vi "fita2_D.vi"() -> ()   [LabVIEW 2014]
uses:
  <vilib>/Analysis/5stat.llb/RMS (DBL).vi
  <vilib>/DAQmx/create/channels.llb/DAQmx Create Channel (AI-Voltage-Basic).vi
  <vilib>/DAQmx/configure/timing.llb/DAQmx Timing (Sample Clock).vi
  <vilib>/DAQmx/read.llb/DAQmx Read (Analog 1D Wfm NChan NSamp).vi
  <vilib>/Waveform/WDTOps.llb/WDT Index Channel DBL.vi
  <vilib>/Utility/file.llb/Write To Spreadsheet File (string).vi
  <vilib>/Analysis/NI_AALPro.lvlib
panel:
  out "CH4":dbl
  out "CH3":dbl
  out "CH2":dbl
  out "CH1":dbl
  out "MIN CH4":bool
  out "MIN CH2":bool
  out "MIN CH1":bool
  out "MIN CH3":bool
  out "MAX CH4":bool
  out "MAX CH3":bool
  out "MAX CH2":bool
  out "MAX CH1":bool
  in  "Temp Max CH2":dbl
  in  "Temp Min CH1":dbl
  in  "Temp Min CH2":dbl
  in  "Temp Max CH3":dbl
  in  "Temp Min CH3":dbl
  in  "Temp Max CH4":dbl
  in  "Temp Min CH4":dbl
  in  "Temp Max CH1":dbl
  in  "Start":bool
  in  "stop":bool
  out "Waveform Chart":T1(graph)
  out "Canals seleccionats":dbl
  in  "Durada adquisicio":dbl
  in  "Temps entre adquisicio":dbl
  in  "Numero de mostres per fer mitja":u32
  in  "Nombre de Canals":string(combo)
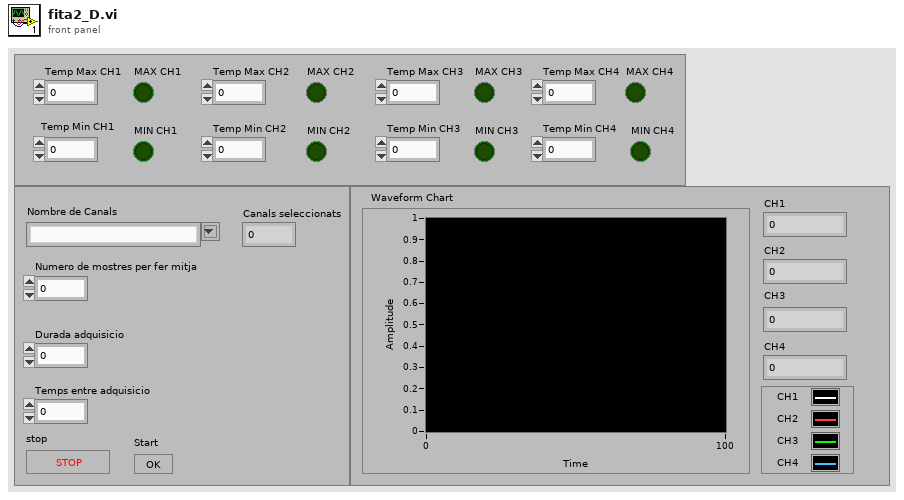
[diagram p1: front panel]
types:
  T1 = cluster{"rms value":dbl, "rms value":dbl, "rms value":dbl, "rms value":dbl}
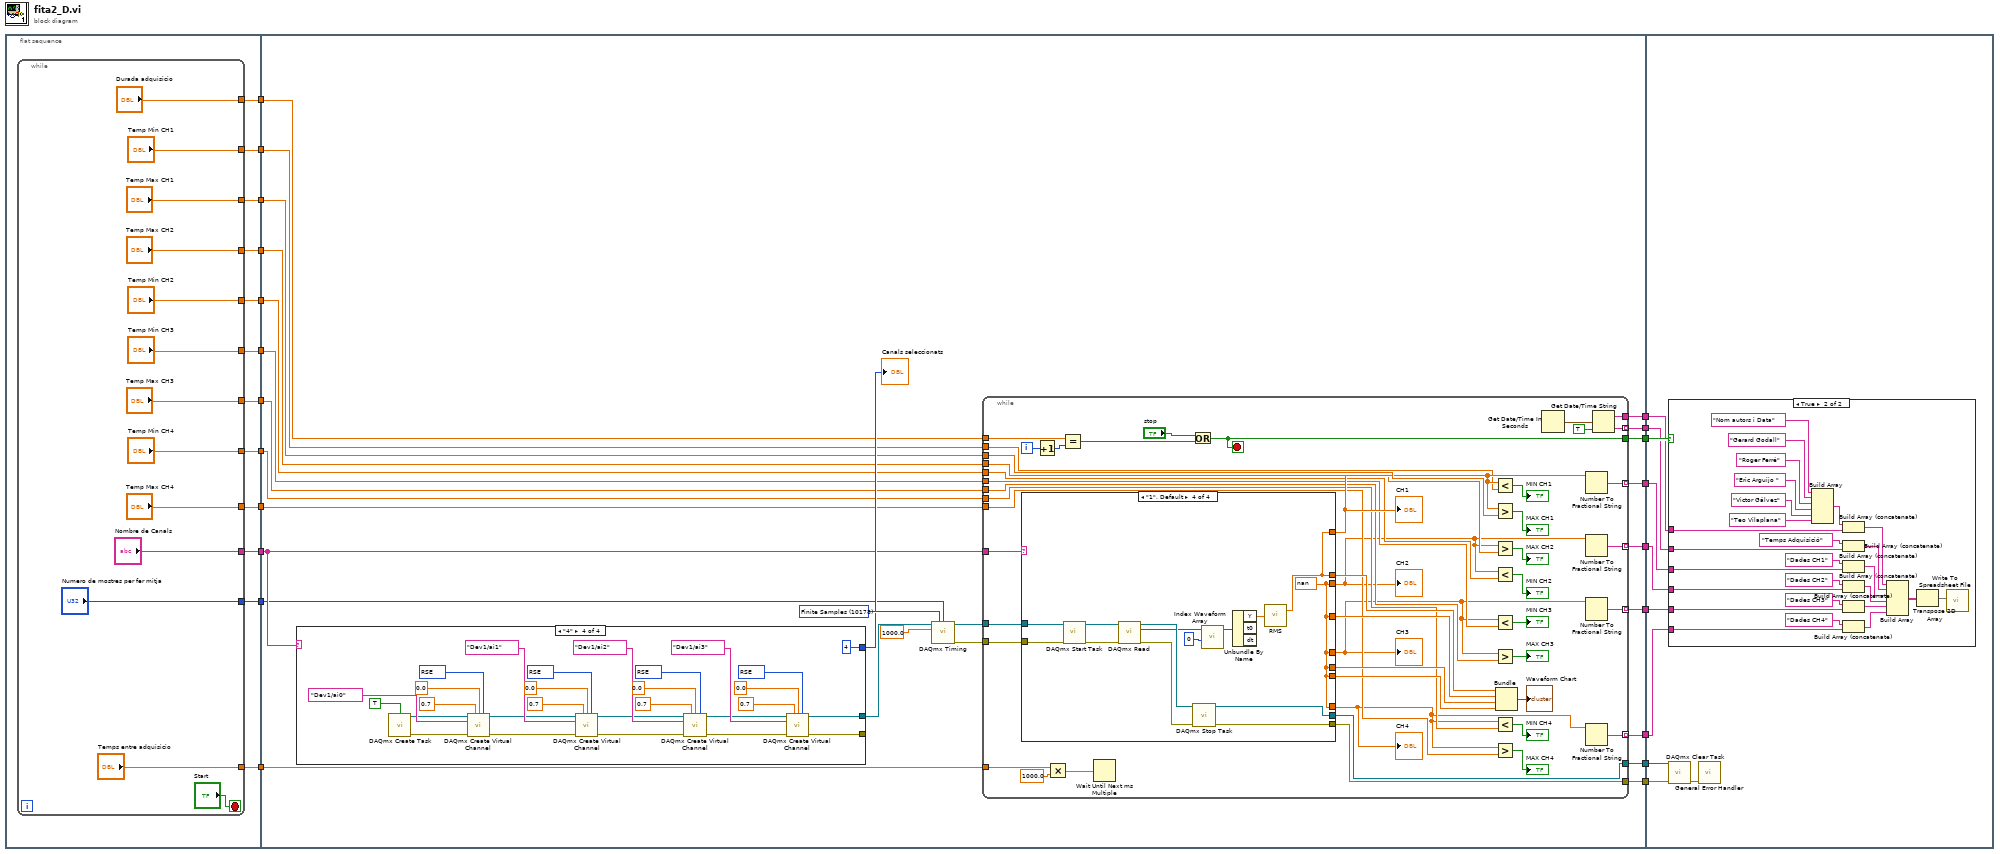
[diagram p0: block diagram]
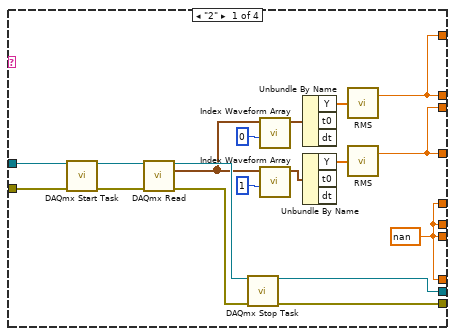
[diagram p2: hidden frame]
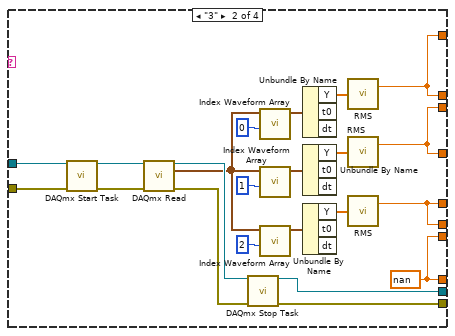
[diagram p3: hidden frame]
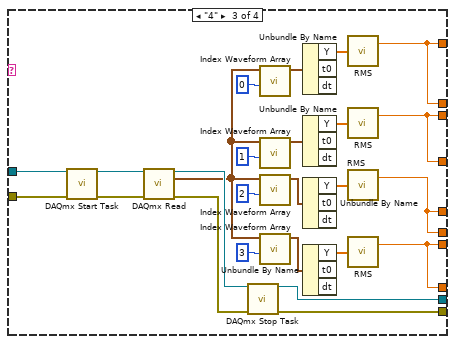
[diagram p4: hidden frame]
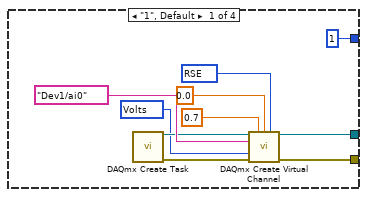
[diagram p5: hidden frame]
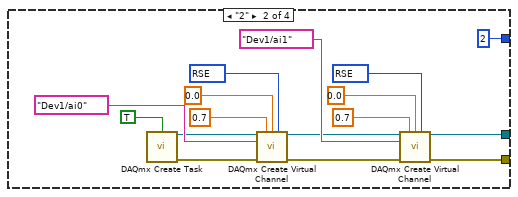
[diagram p6: hidden frame]
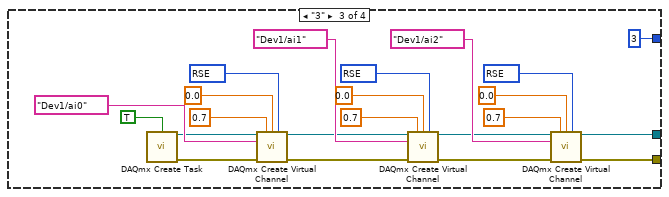
[diagram p7: hidden frame]
diagram:
  n1 = flat-sequence {
    tunnel: [w33] -> w21
    tunnel: [w32] -> w20
    tunnel: [w31] -> w19
    tunnel: [w30] -> w18
    tunnel: [w29] -> w13
    tunnel: [w28] -> w12
    tunnel: [w27] -> w11
    tunnel: [w26] -> w10
    tunnel: [w25] -> w9
    tunnel: [w24] -> w8
    tunnel: [w23] -> w7
    tunnel: [w22] -> w6
    tunnel: w21 -> [w67]
    tunnel: w20 -> [w66]
    tunnel: w19 -> [w65]
    tunnel: w18 -> [w64]
    tunnel: [w63] -> w17
    tunnel: [w62] -> w16
    tunnel: [w61] -> w15
    tunnel: [w60] -> w14
    tunnel: w13 -> [w59]
    tunnel: w12 -> [w58]
    tunnel: w11 -> [w57]
    tunnel: w10 -> [w56]
    tunnel: w9 -> [w55]
    tunnel: w8 -> [w54]
    tunnel: w7 -> [w53]
    tunnel: w6 -> [w52]
    tunnel: [w51] -> w5
    tunnel: [w50] -> w4
    tunnel: [w49] -> w3
    tunnel: [w48] -> w2
    tunnel: [w47] -> w1
    tunnel: w17 -> [w284]
    tunnel: w16 -> [w283]
    tunnel: w15 -> [w282]
    tunnel: w14 -> [w281]
    tunnel: w5 -> [w280]
    tunnel: w4 -> [w279]
    tunnel: w3 -> [w278]
    tunnel: w2 -> [w277]
    tunnel: w1 -> [w276]
    frame #0 {
      n2 = while {
        tunnel: ["Nombre de Canals"] -> w33
        tunnel: ["Durada adquisicio"] -> w32
        tunnel: ["Temps entre adquisicio"] -> w31
        tunnel: ["Numero de mostres per fer mitja"] -> w30
        tunnel: ["Temp Max CH1"] -> w29
        tunnel: ["Temp Min CH1"] -> w28
        tunnel: ["Temp Max CH3"] -> w27
        tunnel: ["Temp Max CH2"] -> w26
        tunnel: ["Temp Max CH4"] -> w25
        tunnel: ["Temp Min CH3"] -> w24
        tunnel: ["Temp Min CH2"] -> w23
        tunnel: ["Temp Min CH4"] -> w22
        stop <- "Start" stop-if-true
      }
    }
    frame #1 {
      w72 = 10178 items=["Finite Samples"=10178, "Continuous Samples"=10123, "Hardware Timed Single Point"=12522] ("sample mode")
      n3 = case shown="\"4\"" w67 {
        tunnel: [w203 w212 w228 w250] -> w73
        tunnel: [w202 w211 w227 w249] -> _
        tunnel: [1 2 3 4] -> w71
        frame "1", Default {
          w200 = 10348 items=["Volts"=10348, "From Custom Scale"=10065] ("units")
          w206 = 10083 items=["default"=-1, "RSE"=10083, "NRSE"=10078, "Differential"=10106, "Pseudodifferential"=12529] ("input terminal configuration")
          n4 = call <vilib>:"DAQmx Create Task.vi"() -> ("task out"=w204:refnum<k21>, "error out"=w205:errorcluster)  [unwired: 14 in]
          n5 = call-poly <vilib>:"DAQmx Create Virtual Channel.vi"("task in"=w204, "maximum value"=0.7, "minimum value"=0.0, "input terminal configuration"=w206, "physical channels"=tag "Dev1/ai0", "units"=w200, "error in"=w205) -> ("task out"=w203:refnum<k21>, "error out"=w202:errorcluster)  [unwired: 7 in]
        }
        frame "2" {
          w215 = 10083 items=["default"=-1, "RSE"=10083, "NRSE"=10078, "Differential"=10106, "Pseudodifferential"=12529] ("input terminal configuration")
          w222 = 10083 items=["default"=-1, "RSE"=10083, "NRSE"=10078, "Differential"=10106, "Pseudodifferential"=12529] ("input terminal configuration")
          n6 = call <vilib>:"DAQmx Create Task.vi"("auto cleanup"=TRUE) -> ("task out"=w220:refnum<k21>, "error out"=w221:errorcluster)  [unwired: 13 in]
          n7 = call-poly <vilib>:"DAQmx Create Virtual Channel.vi"("task in"=w220, "maximum value"=0.7, "minimum value"=0.0, "input terminal configuration"=w222, "physical channels"=tag "Dev1/ai0", "error in"=w221) -> ("task out"=w214:refnum<k21>, "error out"=w213:errorcluster)  [unwired: 8 in]
          n8 = call-poly <vilib>:"DAQmx Create Virtual Channel.vi"("task in"=w214, "maximum value"=0.7, "minimum value"=0.0, "input terminal configuration"=w215, "physical channels"=tag "Dev1/ai1", "error in"=w213) -> ("task out"=w212:refnum<k21>, "error out"=w211:errorcluster)  [unwired: 8 in]
        }
        frame "3" {
          w231 = 10083 items=["default"=-1, "RSE"=10083, "NRSE"=10078, "Differential"=10106, "Pseudodifferential"=12529] ("input terminal configuration")
          w237 = 10083 items=["default"=-1, "RSE"=10083, "NRSE"=10078, "Differential"=10106, "Pseudodifferential"=12529] ("input terminal configuration")
          w244 = 10083 items=["default"=-1, "RSE"=10083, "NRSE"=10078, "Differential"=10106, "Pseudodifferential"=12529] ("input terminal configuration")
          n9 = call <vilib>:"DAQmx Create Task.vi"("auto cleanup"=TRUE) -> ("task out"=w242:refnum<k21>, "error out"=w243:errorcluster)  [unwired: 13 in]
          n10 = call-poly <vilib>:"DAQmx Create Virtual Channel.vi"("task in"=w242, "maximum value"=0.7, "minimum value"=0.0, "input terminal configuration"=w244, "physical channels"=tag "Dev1/ai0", "error in"=w243) -> ("task out"=w236:refnum<k21>, "error out"=w235:errorcluster)  [unwired: 8 in]
          n11 = call-poly <vilib>:"DAQmx Create Virtual Channel.vi"("task in"=w236, "maximum value"=0.7, "minimum value"=0.0, "input terminal configuration"=w237, "physical channels"=tag "Dev1/ai1", "error in"=w235) -> ("task out"=w230:refnum<k21>, "error out"=w229:errorcluster)  [unwired: 8 in]
          n12 = call-poly <vilib>:"DAQmx Create Virtual Channel.vi"("task in"=w230, "maximum value"=0.7, "minimum value"=0.0, "input terminal configuration"=w231, "physical channels"=tag "Dev1/ai2", "error in"=w229) -> ("task out"=w228:refnum<k21>, "error out"=w227:errorcluster)  [unwired: 8 in]
        }
        frame "4" {
          w253 = 10083 items=["default"=-1, "RSE"=10083, "NRSE"=10078, "Differential"=10106, "Pseudodifferential"=12529] ("input terminal configuration")
          w259 = 10083 items=["default"=-1, "RSE"=10083, "NRSE"=10078, "Differential"=10106, "Pseudodifferential"=12529] ("input terminal configuration")
          w265 = 10083 items=["default"=-1, "RSE"=10083, "NRSE"=10078, "Differential"=10106, "Pseudodifferential"=12529] ("input terminal configuration")
          w272 = 10083 items=["default"=-1, "RSE"=10083, "NRSE"=10078, "Differential"=10106, "Pseudodifferential"=12529] ("input terminal configuration")
          n13 = call <vilib>:"DAQmx Create Task.vi"("auto cleanup"=TRUE) -> ("task out"=w270:refnum<k21>, "error out"=w271:errorcluster)  [unwired: 13 in]
          n14 = call-poly <vilib>:"DAQmx Create Virtual Channel.vi"("task in"=w270, "maximum value"=0.7, "minimum value"=0.0, "input terminal configuration"=w272, "physical channels"=tag "Dev1/ai0", "error in"=w271) -> ("task out"=w264:refnum<k21>, "error out"=w263:errorcluster)  [unwired: 8 in]
          n15 = call-poly <vilib>:"DAQmx Create Virtual Channel.vi"("task in"=w264, "maximum value"=0.7, "minimum value"=0.0, "input terminal configuration"=w265, "physical channels"=tag "Dev1/ai1", "error in"=w263) -> ("task out"=w258:refnum<k21>, "error out"=w257:errorcluster)  [unwired: 8 in]
          n16 = call-poly <vilib>:"DAQmx Create Virtual Channel.vi"("task in"=w258, "maximum value"=0.7, "minimum value"=0.0, "input terminal configuration"=w259, "physical channels"=tag "Dev1/ai2", "error in"=w257) -> ("task out"=w252:refnum<k21>, "error out"=w251:errorcluster)  [unwired: 8 in]
          n17 = call-poly <vilib>:"DAQmx Create Virtual Channel.vi"("task in"=w252, "maximum value"=0.7, "minimum value"=0.0, "input terminal configuration"=w253, "physical channels"=tag "Dev1/ai3", "error in"=w251) -> ("task out"=w250:refnum<k21>, "error out"=w249:errorcluster)  [unwired: 8 in]
        }
      }
      "Canals seleccionats" <- w71
      n18 = call-poly <vilib>:"DAQmx Timing.vi"("task/channels in"=w73, "sample mode"=w72, "samples per channel"=w64, "rate"=1000.0) -> ("task out"=w69:refnum<k21>, "error out"=w68:errorcluster)  [unwired: 10 in]
      n19 = while {
        tunnel: w65 -> [w118]
        tunnel: w67 -> [w117]
        tunnel: w69 -> [w116]
        tunnel: w68 -> [w115]
        tunnel: [w114] -> w63
        tunnel: [w113] -> w62
        tunnel: w66 -> [w104]
        tunnel: [w103] -> w61
        tunnel: [w101] -> w60 mode=indexing
        tunnel: w59 -> [w100]
        tunnel: w58 -> [w96]
        tunnel: w57 -> [w88]
        tunnel: w56 -> [w87]
        tunnel: w55 -> [w86]
        tunnel: w54 -> [w85]
        tunnel: w53 -> [w84]
        tunnel: w52 -> [w83]
        tunnel: [w81] -> w51 mode=indexing
        tunnel: [w79] -> w50 mode=indexing
        tunnel: [w77] -> w49 mode=indexing
        tunnel: [w76] -> w48
        tunnel: [w75] -> w47 mode=indexing
        i -> [w110]
        stop <- w103 stop-if-true
        n20 = case shown="\"1\", Default" w117 {
          tunnel: w116 -> [w127 w146 w168 w191]
          tunnel: w115 -> [w126 w145 w167 w190]
          tunnel: [w125 w144 w166 w189] -> w114
          tunnel: [w124 w143 w165 w188] -> w113
          tunnel: [w123 w141 w164 w187] -> w108
          tunnel: [w122 w140 w163 w186] -> w107
          tunnel: [w121 w142 w162 w186] -> w105
          tunnel: [w121 w139 w161 w186] -> w89
          tunnel: [w123 w141 w164 w187] -> w99
          tunnel: [w122 w140 w163 w186] -> w82
          tunnel: [w121 w142 w162 w186] -> w80
          tunnel: [w121 w139 w161 w186] -> w78
          frame "2" {
            w121 = nan ("rms value")
            n21 = call <vilib>:"DAQmx Start Task.vi"("task/channels in"=w127, "error in"=w126) -> ("task out"=w138:refnum<k21>, "error out"=w137:errorcluster)  [unwired: 12 in]
            n22 = call-poly <vilib>:"DAQmx Read.vi"("task/channels in"=w138, "error in"=w137) -> ("task out"=w135:refnum<k21>, "data"=w128:waveform(dbl)[], "error out"=w136:errorcluster)  [unwired: 11 in]
            n23 = call <vilib>:"DAQmx Stop Task.vi"("task/channels in"=w135, "error in"=w136) -> ("task out"=w125:refnum<k21>, "error out"=w124:errorcluster)  [unwired: 12 in]
            n24 = call-poly <vilib>:"Index Waveform Array.vi"("index"=0, "waveform array"=w128) -> ("waveform"=w130:waveform(dbl))  [unwired: 8 in, 1 out]
            n25 = call-poly <vilib>:"Index Waveform Array.vi"("index"=1, "waveform array"=w128) -> ("waveform"=w133:waveform(dbl))  [unwired: 8 in, 1 out]
            n26 = Unbundle By Name(w130) -> ("Y"=w129:dbl[])  [unwired: 2 out]
            n27 = Unbundle By Name(w133) -> ("Y"=w132:dbl[])  [unwired: 2 out]
            n28 = call-poly <vilib>:"RMS.vi"("X"=w129) -> ("rms value"=w123:dbl)  [unwired: 1 out]
            n29 = call-poly <vilib>:"RMS.vi"("X"=w132) -> ("rms value"=w122:dbl)  [unwired: 1 out]
          }
          frame "3" {
            w139 = nan ("rms value")
            n30 = call <vilib>:"DAQmx Start Task.vi"("task/channels in"=w146, "error in"=w145) -> ("task out"=w160:refnum<k21>, "error out"=w159:errorcluster)  [unwired: 12 in]
            n31 = call-poly <vilib>:"DAQmx Read.vi"("task/channels in"=w160, "error in"=w159) -> ("task out"=w157:refnum<k21>, "data"=w147:waveform(dbl)[], "error out"=w158:errorcluster)  [unwired: 11 in]
            n32 = call <vilib>:"DAQmx Stop Task.vi"("task/channels in"=w157, "error in"=w158) -> ("task out"=w144:refnum<k21>, "error out"=w143:errorcluster)  [unwired: 12 in]
            n33 = call-poly <vilib>:"Index Waveform Array.vi"("index"=0, "waveform array"=w147) -> ("waveform"=w152:waveform(dbl))  [unwired: 8 in, 1 out]
            n34 = call-poly <vilib>:"Index Waveform Array.vi"("index"=1, "waveform array"=w147) -> ("waveform"=w149:waveform(dbl))  [unwired: 8 in, 1 out]
            n35 = call-poly <vilib>:"Index Waveform Array.vi"("index"=2, "waveform array"=w147) -> ("waveform"=w155:waveform(dbl))  [unwired: 8 in, 1 out]
            n36 = Unbundle By Name(w152) -> ("Y"=w151:dbl[])  [unwired: 2 out]
            n37 = Unbundle By Name(w149) -> ("Y"=w148:dbl[])  [unwired: 2 out]
            n38 = Unbundle By Name(w155) -> ("Y"=w154:dbl[])  [unwired: 2 out]
            n39 = call-poly <vilib>:"RMS.vi"("X"=w151) -> ("rms value"=w141:dbl)  [unwired: 1 out]
            n40 = call-poly <vilib>:"RMS.vi"("X"=w148) -> ("rms value"=w140:dbl)  [unwired: 1 out]
            n41 = call-poly <vilib>:"RMS.vi"("X"=w154) -> ("rms value"=w142:dbl)  [unwired: 1 out]
          }
          frame "4" {
            n42 = call <vilib>:"DAQmx Start Task.vi"("task/channels in"=w168, "error in"=w167) -> ("task out"=w185:refnum<k21>, "error out"=w184:errorcluster)  [unwired: 12 in]
            n43 = call-poly <vilib>:"DAQmx Read.vi"("task/channels in"=w185, "error in"=w184) -> ("task out"=w182:refnum<k21>, "data"=w169:waveform(dbl)[], "error out"=w183:errorcluster)  [unwired: 11 in]
            n44 = call <vilib>:"DAQmx Stop Task.vi"("task/channels in"=w182, "error in"=w183) -> ("task out"=w166:refnum<k21>, "error out"=w165:errorcluster)  [unwired: 12 in]
            n45 = call-poly <vilib>:"Index Waveform Array.vi"("index"=0, "waveform array"=w169) -> ("waveform"=w174:waveform(dbl))  [unwired: 8 in, 1 out]
            n46 = call-poly <vilib>:"Index Waveform Array.vi"("index"=1, "waveform array"=w169) -> ("waveform"=w171:waveform(dbl))  [unwired: 8 in, 1 out]
            n47 = call-poly <vilib>:"Index Waveform Array.vi"("index"=2, "waveform array"=w169) -> ("waveform"=w180:waveform(dbl))  [unwired: 8 in, 1 out]
            n48 = call-poly <vilib>:"Index Waveform Array.vi"("index"=3, "waveform array"=w169) -> ("waveform"=w177:waveform(dbl))  [unwired: 8 in, 1 out]
            n49 = Unbundle By Name(w174) -> ("Y"=w173:dbl[])  [unwired: 2 out]
            n50 = Unbundle By Name(w171) -> ("Y"=w170:dbl[])  [unwired: 2 out]
            n51 = Unbundle By Name(w180) -> ("Y"=w179:dbl[])  [unwired: 2 out]
            n52 = Unbundle By Name(w177) -> ("Y"=w176:dbl[])  [unwired: 2 out]
            n53 = call-poly <vilib>:"RMS.vi"("X"=w173) -> ("rms value"=w164:dbl)  [unwired: 1 out]
            n54 = call-poly <vilib>:"RMS.vi"("X"=w170) -> ("rms value"=w163:dbl)  [unwired: 1 out]
            n55 = call-poly <vilib>:"RMS.vi"("X"=w179) -> ("rms value"=w162:dbl)  [unwired: 1 out]
            n56 = call-poly <vilib>:"RMS.vi"("X"=w176) -> ("rms value"=w161:dbl)  [unwired: 1 out]
          }
          frame "1", Default {
            w186 = nan ("rms value")
            n57 = call <vilib>:"DAQmx Start Task.vi"("task/channels in"=w191, "error in"=w190) -> ("task out"=w199:refnum<k21>, "error out"=w198:errorcluster)  [unwired: 12 in]
            n58 = call-poly <vilib>:"DAQmx Read.vi"("task/channels in"=w199, "error in"=w198) -> ("task out"=w196:refnum<k21>, "data"=w192:waveform(dbl)[], "error out"=w197:errorcluster)  [unwired: 11 in]
            n59 = call <vilib>:"DAQmx Stop Task.vi"("task/channels in"=w196, "error in"=w197) -> ("task out"=w189:refnum<k21>, "error out"=w188:errorcluster)  [unwired: 12 in]
            n60 = call-poly <vilib>:"Index Waveform Array.vi"("index"=0, "waveform array"=w192) -> ("waveform"=w194:waveform(dbl))  [unwired: 8 in, 1 out]
            n61 = Unbundle By Name(w194) -> ("Y"=w193:dbl[])  [unwired: 2 out]
            n62 = call-poly <vilib>:"RMS.vi"("X"=w193) -> ("rms value"=w187:dbl)  [unwired: 1 out]
          }
        }
        "CH1" <- w99
        "CH2" <- w82
        "CH3" <- w80
        "CH4" <- w78
        n63 = Increment(x=w110) -> (x+1=w109:i32)
        n64 = Multiply(x=w118, y=1000.0) -> (x*y=w119:dbl)
        n65 = Equal?(x=w104, y=w109) -> (x = y?=w111:bool)
        n66 = Wait Until Next ms Multiple(millisecond multiple=w119) -> ()  [unwired: 1 out]
        n67 = Or(x="stop", y=w111) -> (x .or. y?=w103:bool)
        n68 = Less?(x=w99, y=w96) -> (x < y?=→"MIN CH1":bool)
        n69 = Greater?(x=w99, y=w100) -> (0:→"MAX CH1":bool)
        n70 = Greater?(x=w82, y=w87) -> (0:→"MAX CH2":bool)
        n71 = Less?(x=w82, y=w84) -> (x < y?=→"MIN CH2":bool)
        n72 = Less?(x=w80, y=w85) -> (x < y?=→"MIN CH3":bool)
        n73 = Greater?(x=w80, y=w88) -> (0:→"MAX CH3":bool)
        n74 = Less?(x=w78, y=w83) -> (x < y?=→"MIN CH4":bool)
        n75 = Greater?(x=w78, y=w86) -> (0:→"MAX CH4":bool)
        n76 = Bundle("rms value"=w108, "rms value"=w107, "rms value"=w105, "rms value"=w89) -> (→"Waveform Chart":T1)  [unwired: 1 in]
        n77 = Get Date/Time In Seconds() -> (seconds since 1Jan1904=w102:timestamp)
        n78 = Number To Fractional String(number=w99) -> (F-format string=w101:string)  [unwired: 3 in]
        n79 = Number To Fractional String(number=w82) -> (F-format string=w81:string)  [unwired: 3 in]
        n80 = Number To Fractional String(number=w80) -> (F-format string=w79:string)  [unwired: 3 in]
        n81 = Number To Fractional String(number=w78) -> (F-format string=w77:string)  [unwired: 3 in]
        n82 = Get Date/Time String(seconds (now)=w102, want seconds? (F)=TRUE) -> (date string=w76:string, time string=w75:string)  [unwired: 1 in]
      }
    }
    frame #2 {
      n83 = case shown="True" w282 {
        tunnel: w281 -> [_ w296]
        tunnel: w280 -> [_ w292]
        tunnel: w279 -> [_ w286]
        tunnel: w278 -> [_ w287]
        tunnel: w276 -> [_ w299]
        tunnel: w277 -> [_ w298]
        frame False {
        }
        frame True {
          n84 = Build Array("Nom autors i Data" ("element"), "Gerard Godall", "Roger Ferré" ("element"), "Eric Arguijo " ("element"), "Victor Gálvez" ("element"), "Teo Vilaplana" ("element")) -> (w305:string[])
          n85 = Build Array (concatenate)(w305, w298) -> (w304:string[])
          n86 = Build Array (concatenate)("Temps Adquisició", w299) -> (w300:string[])
          n87 = Build Array (concatenate)("Dades CH1", w296) -> (w295:string[])
          n88 = Build Array (concatenate)("Dades CH2", w292) -> (w294:string[])
          n89 = Build Array (concatenate)("Dades CH3", w286) -> (w291:string[])
          n90 = Build Array (concatenate)("Dades CH4", w287) -> (w290:string[])
          n91 = Build Array(w304, w300, w295, w294, w291, w290) -> (w311:string[][])
          n92 = Transpose 2D Array(2D array=w311) -> (transposed array=w303:string[][])
          n93 = call-poly <vilib>:"Write To Spreadsheet File.vi"("2D data"=w303) -> ()  [unwired: 7 in, 1 out]
        }
      }
      n94 = call <vilib>:"DAQmx Clear Task.vi"("task in"=w284, "error in"=w283) -> ("error out"=w285:errorcluster)  [unwired: 13 in]
      n95 = call <vilib>:"General Error Handler.vi"("error in (no error)"=w285) -> ()  [unwired: 10 in, 5 out]
    }
  }
